vi "Horizontal Panel.vi"() -> ()   [LabVIEW 2013, in "PanelDataNode.lvclass"]
uses:
  PanelDataNode.lvclass
  PanelObject/PanelObject.lvclass
  Split Mode.ctl
  PanelLinkNode/PanelLinkNode.lvclass
panel:
  in  "Node*":refnum<data-value>
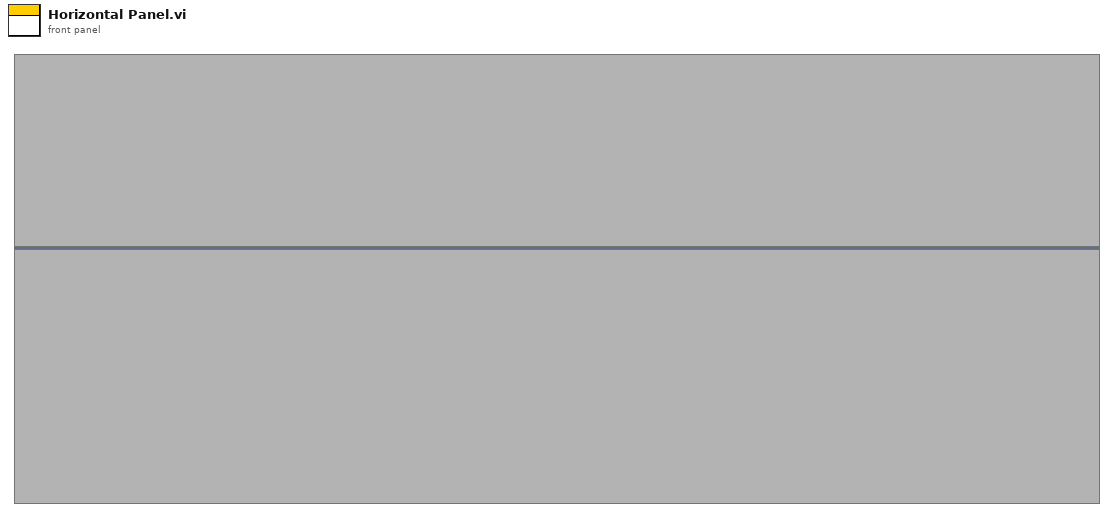
[diagram p1: front panel]
types:
  T1 = typedef "PanelDataNode.lvclass/Split Mode.ctl" = enum16{"Horizontal(up)", "Vertical(left)", "Horizontal(down)", "Vertical(right)"}
  T2 = cluster{"ChildNode*":refnum<data-value>, "Split Mode":T1}
  T3 = cluster{"ChildNode*":refnum<data-value>, "VI*":refnum<vi>}
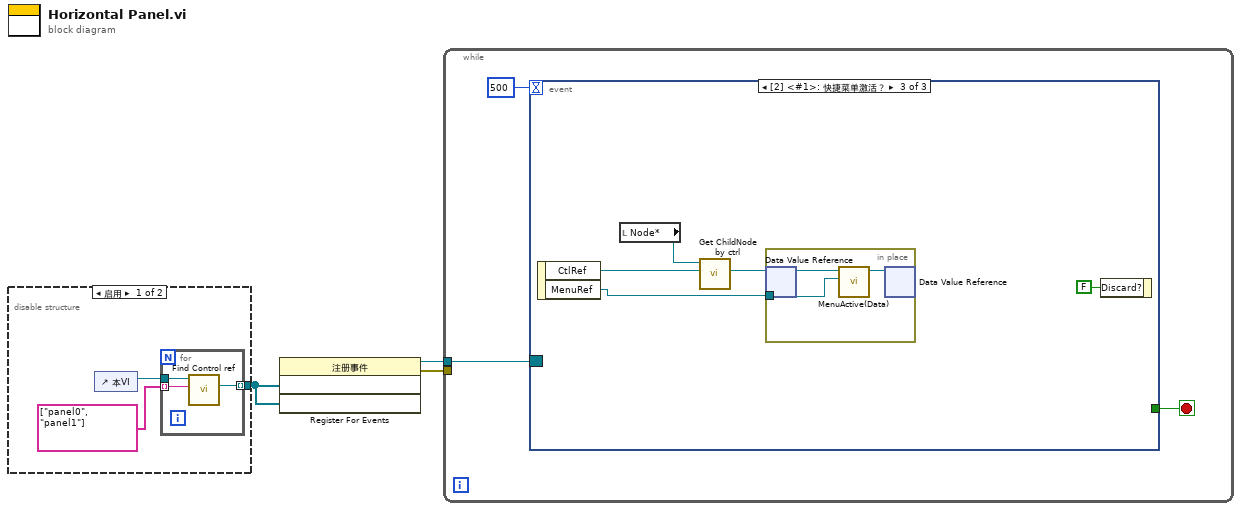
[diagram p0: block diagram]
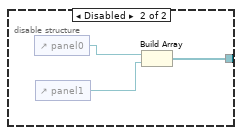
[diagram p2: hidden frame]
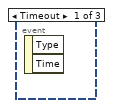
[diagram p3: hidden frame]
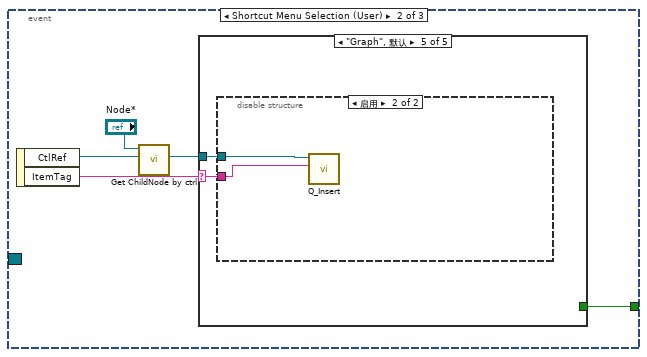
[diagram p4: hidden frame]
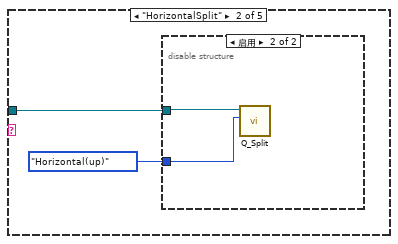
[diagram p6: hidden frame]
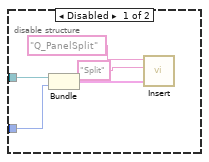
[diagram p7: hidden frame]
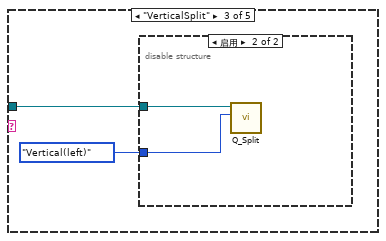
[diagram p8: hidden frame]
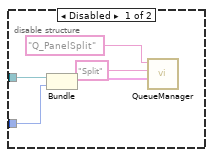
[diagram p9: hidden frame]
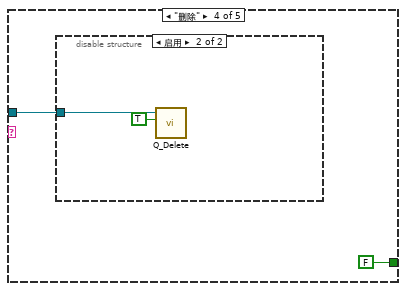
[diagram p10: hidden frame]
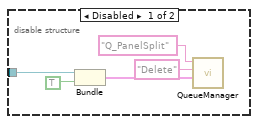
[diagram p11: hidden frame]
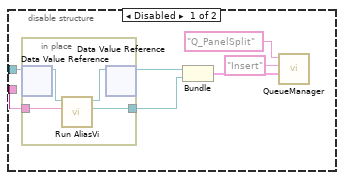
[diagram p12: hidden frame]
diagram:
  n1 = disable-structure shown="启用" {
    disable-tunnel: [w4 w10] -> w2
    frame Enabled {
      n2 = control-ref of="本VI"() -> (w6:refnum<vi>)
      n3 = for {
        tunnel: w6 -> [w9]
        tunnel: string[] ["panel0", "panel1"] -> [w8] mode=indexing
        tunnel: [w7] -> w4 mode=indexing
        n4 = call "Find Control ref.vi"("control name"=w8, "panelvi*"=w9) -> ("ctrl*"=w7:refnum<vi>)  [unwired: 7 in, 2 out]
      }
    }
    frame Disabled {
      n5 = control-ref of="panel0"() -> (w12:refnum<vi>)
      n6 = control-ref of="panel1"() -> (w11:refnum<vi>)
      n7 = Build Array(w12, w11) -> (w10:refnum<vi>[])
    }
  }
  n8 = register-events(w2, w2) -> (reference out=w3:refnum<event-registration>, error out=w1:errorcluster)  [unwired: 2 in]
  n9 = while {
    tunnel: w3 -> [w14]
    tunnel: w1 -> [_]
    stop <- w13 stop-if-true
    n10 = event shown="[2] <#1>: 快捷菜单激活？" {
      selector: w14 -> [_ _ _]
      dyn-events: _ -> [_ _ _]
      timeout: 500 -> [_ _ _]
      tunnel: [_ w16 _] -> w13
      event Timeout {
        n11 = event-data() -> ()  [unwired: 1 in, 2 out]
      }
      event Shortcut Menu Selection (User) {
        n12 = event-data() -> ("CtlRef"=w20:refnum<vi>, "ItemTag"=w17:string)  [unwired: 1 in]
        n13 = call "Get ChildNode by ctrl.vi"("ctr*"=w20, "Node*"="Node*") -> ("ChildNode*"=w18:refnum<data-value>)  [unwired: 8 in, 1 out]
        n14 = case shown="\"Graph\", 默认" w17 {
          selector: w17 -> [_ _ _ _ w49]
          tunnel: w18 -> [_ w22 w30 w39 w48]
          tunnel: [_ _ _ FALSE _] -> w16
          frame "假" {
          }
          frame "HorizontalSplit" {
            n15 = disable-structure shown="启用" {
              disable-tunnel: w22 -> [w27 w29]
              disable-tunnel: Split_Mode."Horizontal(up)" ("Split Mode") -> [w26 w28]
              frame Disabled {
                n16 = Bundle("ChildNode*"=w27, "Split Mode"=w26) -> (w25:T2)  [unwired: 1 in]
                n17 = call "Insert.vi"("Data"=w25, "Event"="Split", "QueueName"="Q_PanelSplit") -> ()  [unwired: 7 in, 2 out]
              }
              frame Enabled {
                n18 = call "Q_Split.vi"("Split Mode"=w28, "ChildNode*"=w29) -> ()  [unwired: 9 in, 1 out]
              }
            }
          }
          frame "VerticalSplit" {
            n19 = disable-structure shown="启用" {
              disable-tunnel: Split_Mode."Vertical(left)" ("Split Mode") -> [w36 w38]
              disable-tunnel: w30 -> [w35 w37]
              frame Disabled {
                n20 = Bundle("ChildNode*"=w35, "Split Mode"=w36) -> (w32:T2)  [unwired: 1 in]
                n21 = call-poly "QueueManager.vi"("Data"=w32, "Event"="Split", "QueueName"="Q_PanelSplit") -> ()  [unwired: 7 in, 2 out]
              }
              frame Enabled {
                n22 = call "Q_Split.vi"("Split Mode"=w38, "ChildNode*"=w37) -> ()  [unwired: 9 in, 1 out]
              }
            }
          }
          frame "删除" {
            n23 = disable-structure shown="启用" {
              disable-tunnel: w39 -> [w45 w47]
              frame Disabled {
                n24 = Bundle("ChildNode*"=w45, TRUE) -> (w44:cluster{"ChildNode*":refnum<data-value>, bool})  [unwired: 1 in]
                n25 = call-poly "QueueManager.vi"("Data"=w44, "Event"="Delete", "QueueName"="Q_PanelSplit") -> ()  [unwired: 7 in, 2 out]
              }
              frame Enabled {
                n26 = call "Q_Delete.vi"("CloseVI?(T)"=TRUE, "ChildNode*"=w47) -> ()  [unwired: 9 in, 1 out]
              }
            }
          }
          frame "Graph", Default {
            n27 = disable-structure shown="启用" {
              disable-tunnel: w49 -> [w53 w61]
              disable-tunnel: w48 -> [w52 w62]
              frame Disabled {
                n28 = in-place {
                  in-place-border: w53 -> [w60]
                  in-place-border: [w57] -> w50
                  n29 = in-place-dvr #1(w52) -> (w59:refnum<class "PanelDataNode.lvclass">)  [unwired: 1 out]
                  n30 = call-dynamic "Run AliasVi.vi"("Vi Alias"=w60, "PanelDataNode 输入"=w59) -> ("VI*"=w57:refnum<vi>, "PanelDataNode 输出"=w58:refnum<class "PanelDataNode.lvclass">)  [unwired: 7 in, 1 out]
                  n31 = in-place-dvr #1(w58) -> (w51:refnum<data-value>)  [unwired: 1 out]
                }
                n32 = Bundle("ChildNode*"=w51, "VI*"=w50) -> (w56:T3)  [unwired: 1 in]
                n33 = call-poly "QueueManager.vi"("Data"=w56, "Event"="Insert", "QueueName"="Q_PanelSplit") -> ()  [unwired: 7 in, 2 out]
              }
              frame Enabled {
                n34 = call "Q_Insert.vi"("Vi Alias"=w61, "ChildNode*"=w62) -> ()  [unwired: 9 in, 1 out]
              }
            }
          }
        }
      }
      event Shortcut Menu Activation? {
        n35 = event-data() -> ("CtlRef"=w67:refnum<vi>, "MenuRef"=w64:refnum<k9>)  [unwired: 1 in]
        n36 = local read "Node*"() -> (w66:refnum<data-value>)
        n37 = call "Get ChildNode by ctrl.vi"("ctr*"=w67, "Node*"=w66) -> ("ChildNode*"=w65:refnum<data-value>)  [unwired: 8 in, 1 out]
        n38 = in-place {
          in-place-border: w64 -> [w69]
          n39 = in-place-dvr #2(w65) -> (w70:refnum<class "PanelDataNode.lvclass">)  [unwired: 1 out]
          n40 = call-dynamic "MenuActive(Data).vi"("菜单引用"=w69, "PanelDataNode 输入"=w70) -> ("PanelDataNode 输出"=w68:refnum<class "PanelDataNode.lvclass">)  [unwired: 7 in, 2 out]
          n41 = in-place-dvr #2(w68) -> ()  [unwired: 2 out]
        }
        n42 = event-data("Discard?"=FALSE ("放弃？")) -> ()  [unwired: 1 in, 1 out]
      }
    }
  }
